vi "SimpleTestTreeConfig.vi"(8 "error in":errorcluster) -> (0 "error out":errorcluster, 2 "summary":T1[](array[typedef]), 3 "Data Value Reference out":T2)   [LabVIEW 2014, in "NISE_CEF_Tests.lvlib"]
uses:
  NISE_CEF_Tests.lvlib
  Trunk/Configuration Framework/Node/NodeRef.ctl
  Trunk/Configuration Framework/Node/NISE_CEF_Node.lvclass
  Trunk/Configuration Framework/Node/Summary.ctl
  Trunk/ProjectTemplates/Source/Configuration Editor Framework/Classes/cRIO/cRIO.lvclass
  Trunk/ProjectTemplates/Source/Configuration Editor Framework/Classes/Group/Group.lvclass
  Trunk/ProjectTemplates/Source/Configuration Editor Framework/Classes/Voltage/Voltage.lvclass
  Trunk/Configuration Framework/NISE_CEF_TreeControl.lvlib
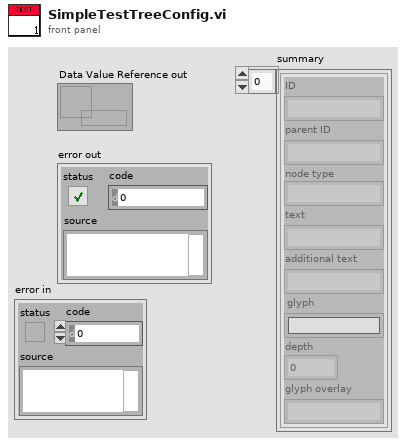
[diagram p1: front panel]
types:
  T1 = typedef "NISE_CEF_Node.lvclass/Summary.ctl" = cluster{"ID":string, "parent ID":string, "node type":string, "text":string, "additional text":string, "glyph":string, "depth":i32, "glyph overlay":string}
  T2 = typedef "NISE_CEF_Node.lvclass/NodeRef.ctl" = refnum<data-value>
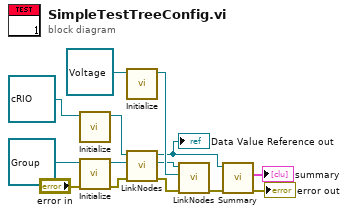
[diagram p0: block diagram]
diagram:
  n1 = call-dynamic "Initialize.vi"("cRIO in"=refnum<class "cRIO.lvclass"> refnum ("cRIO.lvclass")) -> ("data value reference"=w10:T2)  [unwired: 8 in, 2 out]
  n2 = call-dynamic "Initialize.vi"("error in"="error in", "group in"=refnum<class "Group.lvclass"> refnum ("Group.lvclass")) -> ("error out"=w1:errorcluster, "data value reference"=w11:T2)  [unwired: 7 in, 1 out]
  n3 = call-dynamic "Initialize.vi"("voltage in"=refnum<class "Voltage.lvclass"> refnum ("Voltage.lvclass")) -> ("data value reference"=w13:T2)  [unwired: 8 in, 2 out]
  n4 = call "LinkNodes.vi"("error in"=w1, "child in"=w11, "parent in"=w10) -> ("error out"=w14:errorcluster, "child out"=w12:T2, "parent out"=w6:T2)  [unwired: 6 in]
  "Data Value Reference out" <- w6
  n5 = call "LinkNodes.vi"("error in"=w14, "child in"=w13, "parent in"=w12) -> ("error out"=w5:errorcluster)  [unwired: 6 in, 2 out]
  n6 = call "Summary.vi"("error in"=w5, "node self ref"=w6) -> ("error out"=→"error out":errorcluster, "summary"=→"summary":T1[])  [unwired: 8 in]
